vi "Write Output Data.vi"(10 "Output Data":T1 {"Step & Direction" min=-32767}, 11 "Logger in":refnum<class "Logger.lvclass">) -> (3 "Logger out":refnum<class "Logger.lvclass">)   [LabVIEW 2013, in "Logger.lvclass"]
uses:
  Logger.lvclass
  Typedefs/OutputData.ctl
  Logger.lvclass/Logger.ctl
  Typedefs/M2AADTTypedefs.lvlib
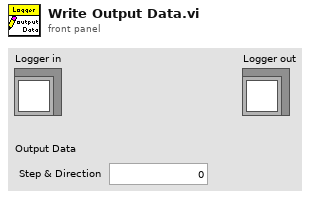
[diagram p1: front panel]
types:
  T1 = typedef "M2AADTTypedefs.lvlib/OutputData.ctl" = cluster{"Step & Direction":i16}
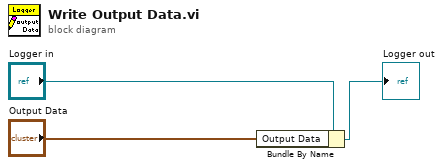
[diagram p0: block diagram]
diagram:
  n1 = Bundle By Name(cluster="Logger in", "Output Data"="Output Data") -> (→"Logger out":refnum<class "Logger.lvclass">)
